vi "Strip Struct Padding.vi"(8 "error in (no error)":errorcluster, 9 "[Sub-Item Type Information]":T1[](array[typedef]), 10 "Byte Stream in":u8[](array[numeric]), 11 "TwinCAT ADS in":refnum<class "TwinCAT ADS.lvclass">) -> (0 "error out":errorcluster, 2 "Data String":string, 3 "TwinCAT ADS out":refnum<class "TwinCAT ADS.lvclass">)   [LabVIEW 2018, in "TwinCAT ADS.lvclass"]
uses:
  TwinCAT ADS.lvclass
  Controls/PLC Sub-Item Type Descriptor.ctl
  Controls/PLC Type.ctl
  Controls/PLC Array Type Descriptor.ctl
  PLC Primitive Byte Stream to Data String.vi/dd5e40b3-f89d-44d0-b911-1f2dc1f1e391.vi
  PLC Primitive Byte Stream to Data String.vi/9a8c356b-cf55-4838-9201-0532b80217b2.vi
  PLC Primitive Byte Stream to Data String.vi/06482052-d1f9-4f29-aca9-908031c6a69f.vi
  PLC Primitive Byte Stream to Data String.vi/b9242781-96b0-446e-9150-452b1084ed54.vi
  PLC Primitive Byte Stream to Data String.vi/5fbe6976-0b86-40a2-b7b6-3748894f0071.vi
  PLC Primitive Byte Stream to Data String.vi/c4de1741-fffd-4fed-ba25-d7b4acbf0555.vi
  PLC Primitive Byte Stream to Data String.vi/20356124-05d2-4a04-a5d1-e69adc4c58c2.vi
  PLC Primitive Byte Stream to Data String.vi/67ddb754-0fbe-43d9-9e61-34d6659124ef.vi
  PLC Primitive Byte Stream to Data String.vi/e3d41cb3-d20e-45e9-8252-e41884a8f4d0.vi
  PLC Primitive Byte Stream to Data String.vi/46ba2a54-cc07-4222-9a0e-bd972edfcef0.vi
  PLC Primitive Byte Stream to Data String.vi/6b416cf7-30dc-48a3-9278-9d800f443678.vi
  PLC Primitive Byte Stream to Data String.vi/5857d013-9824-4299-a2d7-53efdc0d26c5.vi
  PLC Primitive Byte Stream to Data String.vi/006b0e7e-7e80-41f3-be4e-1f3da8479fae.vi
  PLC Primitive Byte Stream to Data String.vi/28d9c90b-5f2a-4c58-95e2-5fc46303b0fd.vi
  PLC Primitive Byte Stream to Data String.vi/99b7bc4a-962e-4818-aa5d-444f23f83b11.vi
  PLC Primitive Byte Stream to Data String.vi/8b7c42c8-9170-4542-8f35-15cbeddc22cb.vi
  PLC Primitive Byte Stream to Data String.vi/65a091fa-0bd2-4a35-ae2b-3fa5e90d1994.vi
  PLC Primitive Byte Stream to Data String.vi/4b7d3a7d-7f1b-46f0-9357-48cb72148c56.vi
  PLC Primitive Byte Stream to Data String.vi/b431183c-2ad5-4c6d-9bfa-a53b18913682.vi
  PLC Primitive Byte Stream to Data String.vi/30c6c28a-53c3-4e33-80b1-b22f521e1f67.vi
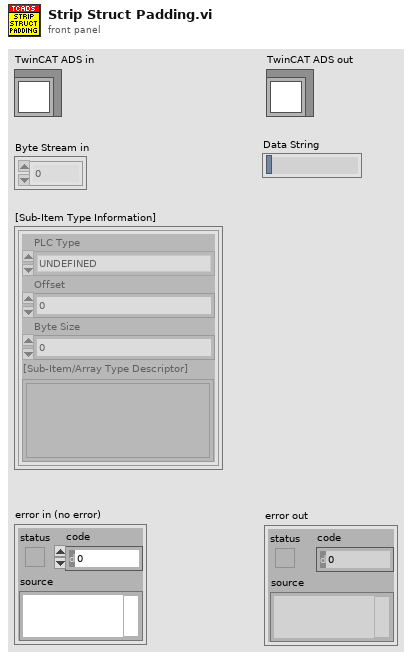
[diagram p1: front panel]
types:
  T1 = typedef "TwinCAT ADS.lvclass/PLC Sub-Item Type Descriptor.ctl" = cluster{"PLC Type":T2, "Offset":i32, "Byte Size":i32, "[Sub-Item/Array Type Descriptor]":variant[]}
  T2 = typedef "TwinCAT ADS.lvclass/PLC Type.ctl" = enum16{"UNDEFINED", "INT", "DINT", "REAL", "LREAL", "SINT", "BYTE", "UINT", "UDINT", "LINT", "ULINT", "STRING", "WSTRING", "BOOL", "TIME", "LTIME", "DATE", "DT", "TOD", "ARRAY", "JAGGED ARRAY", "STRUCT", "FUNCTION BLOCK", "UNION", "POINTER", "USER DEFINED"}
  T3 = typedef "TwinCAT ADS.lvclass/PLC Array Type Descriptor.ctl" = cluster{"Fundamental PLC Type":T2, "Fundamental Type Byte Size":i32, "Item Count":i32, "Dimension Lengths":i32[], "Sub-Item Type Descriptor":variant}
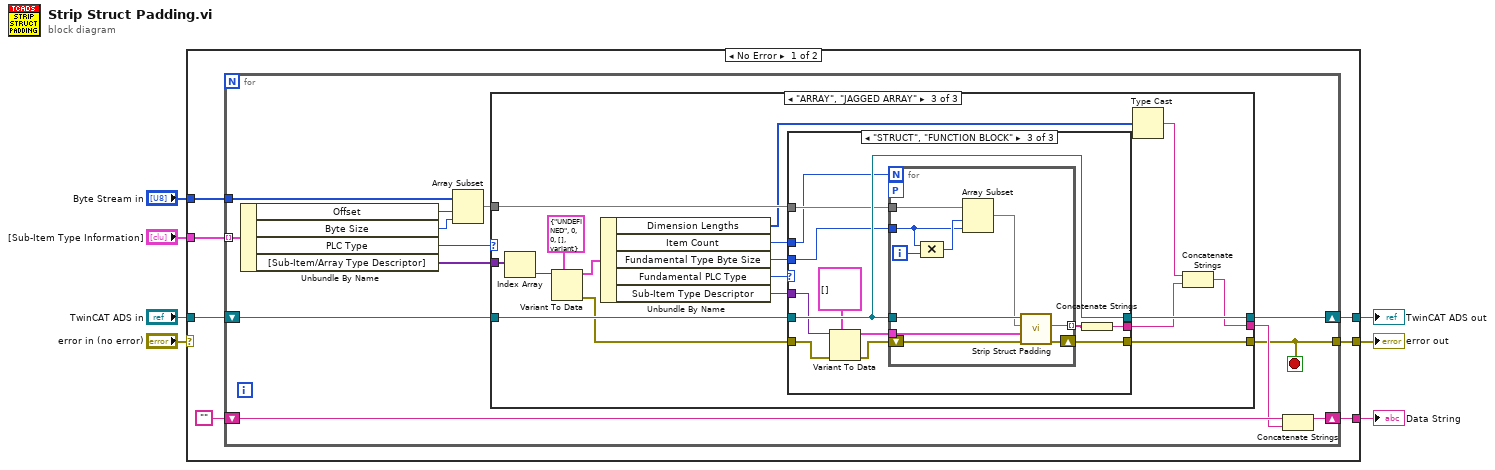
[diagram p0: block diagram]
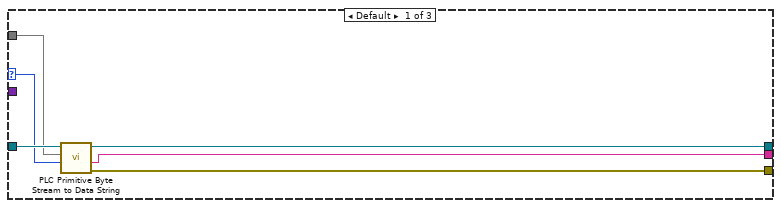
[diagram p2: hidden frame]
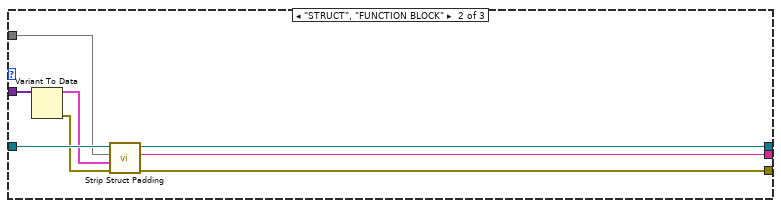
[diagram p3: hidden frame]
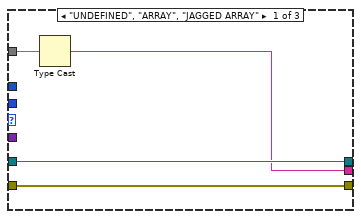
[diagram p4: hidden frame]
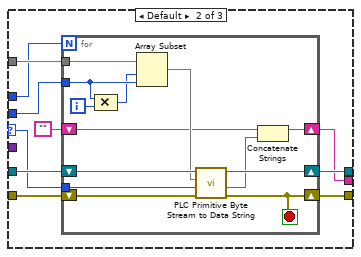
[diagram p5: hidden frame]
diagram:
  n1 = case shown="No Error" "error in (no error)" {
    selector: "error in (no error)" -> [_ w109]
    tunnel: "[Sub-Item Type Information]" -> [w14 _]
    tunnel: "Byte Stream in" -> [w13 _]
    tunnel: [w11 _] -> w5
    tunnel: [w10 w109] -> w4
    tunnel: "TwinCAT ADS in" -> [w9 w108]
    tunnel: [w8 w108] -> w1
    frame No Error {
      n2 = for {
        tunnel: w14 -> [w27] mode=indexing
        shift-right: [w20] -> w11
        shift-left: "" -> [w21]
        tunnel: [w17] -> w10
        tunnel: w13 -> [w26]
        shift-right: [w16] -> w8
        shift-left: w9 -> [w15]
        stop <- w17 stop-if-true
        n3 = Unbundle By Name(w27) -> ("Offset"=w25:i32, "Byte Size"=w24:i32, "PLC Type"=w22:T2, "[Sub-Item/Array Type Descriptor]"=w18:variant[])
        n4 = Array Subset(array=w26, index=w25, length=w24) -> (w23:u8[])
        n5 = case shown="\"ARRAY\", \"JAGGED ARRAY\"" w22 {
          selector: w22 -> [w32 _ _]
          tunnel: w23 -> [w31 w35 w51]
          tunnel: [w28 w37 w42] -> w19
          tunnel: w18 -> [_ w39 w58]
          tunnel: [w30 w38 w45] -> w17
          tunnel: [w29 w34 w46] -> w16
          tunnel: w15 -> [w33 w41 w54]
          frame Default {
            n6 = call "PLC Primitive Byte Stream to Data String.vi"("PLC Type"=w32, "Byte Stream"=w31, "TwinCAT ADS in"=w33) -> ("error out"=w30:errorcluster, "Data String"=w28:string, "TwinCAT ADS out"=w29:refnum<class "TwinCAT ADS.lvclass">)  [unwired: 5 in, 1 out]
          }
          frame "STRUCT", "FUNCTION BLOCK" {
            n7 = Variant To Data(Variant=w39) -> (data=w36:T1[], error out=w40:errorcluster)  [unwired: 2 in]
            n8 = call "Strip Struct Padding.vi"("error in (no error)"=w40, "[Sub-Item Type Information]"=w36, "Byte Stream in"=w35, "TwinCAT ADS in"=w41) -> ("error out"=w38:errorcluster, "Data String"=w37:string, "TwinCAT ADS out"=w34:refnum<class "TwinCAT ADS.lvclass">)  [unwired: 5 in]
          }
          frame "ARRAY", "JAGGED ARRAY" {
            n9 = Index Array(array=w58) -> (element=w57:variant)  [unwired: 1 in]
            n10 = Variant To Data(type=T3 {"Fundamental PLC Type"=enum."UNDEFINED", "Fundamental Type Byte Size"=0, "Item Count"=0, "Dimension Lengths"=[], "Sub-Item Type Descriptor"=variant} ("Array Information"), Variant=w57) -> (data=w55:T3, error out=w52:errorcluster)  [unwired: 1 in]
            n11 = Unbundle By Name(w55) -> ("Dimension Lengths"=w47:i32[], "Item Count"=w48:i32, "Fundamental Type Byte Size"=w49:i32, "Fundamental PLC Type"=w50:T2, "Sub-Item Type Descriptor"=w53:variant)
            n12 = case shown="\"STRUCT\", \"FUNCTION BLOCK\"" w50 {
              selector: w50 -> [_ w66 _]
              tunnel: w52 -> [w61 w67 w92]
              tunnel: w54 -> [w62 w71 w97]
              tunnel: w51 -> [w60 w72 w95]
              tunnel: [w61 w65 w96] -> w45
              tunnel: [w62 w64 w97] -> w46
              tunnel: w53 -> [_ _ w91]
              tunnel: w48 -> [_ w70 w94]
              tunnel: w49 -> [_ w69 w93]
              tunnel: [w59 w63 w86] -> w44
              frame "UNDEFINED", "ARRAY", "JAGGED ARRAY" {
                n13 = Type Cast(x=w60) -> (*(type *) &x=w59:string)  [unwired: 1 in]
              }
              frame Default {
                n14 = for {
                  N: w70 -> [_]
                  shift-right: [w77] -> w64
                  shift-left: w71 -> [w81]
                  tunnel: w66 -> [w79]
                  tunnel: w69 -> [w83]
                  shift-right: [w76] -> w65
                  shift-left: w67 -> [w80]
                  tunnel: w72 -> [w85]
                  shift-right: [w74] -> w63
                  shift-left: "" -> [w73]
                  i -> [w84]
                  stop <- w76 stop-if-true
                  n15 = Compound Arithmetic op=MULTIPLY(w83, w84) -> (w82:i32)
                  n16 = Array Subset(array=w85, index=w82, length=w83) -> (w78:u8[])
                  n17 = call "PLC Primitive Byte Stream to Data String.vi"("error in (no error)"=w80, "PLC Type"=w79, "Byte Stream"=w78, "TwinCAT ADS in"=w81) -> ("error out"=w76:errorcluster, "Data String"=w75:string, "TwinCAT ADS out"=w77:refnum<class "TwinCAT ADS.lvclass">)  [unwired: 4 in, 1 out]
                  n18 = Concatenate Strings(w73, w75) -> (w74:string)
                }
              }
              frame "STRUCT", "FUNCTION BLOCK" {
                n19 = Variant To Data(error in=w92, type=T1[] [] ("[Sub-Item Type Information]"), Variant=w91) -> (data=w88:T1[], error out=w90:errorcluster)
                n20 = for {
                  N: w94 -> [_]
                  tunnel: w93 -> [w104]
                  tunnel: w88 -> [w103]
                  shift-right: [w99] -> w96
                  shift-left: w90 -> [w101]
                  tunnel: w95 -> [w106]
                  workers-P: _ -> [_]
                  tunnel: w97 -> [w102]
                  tunnel: [w100] -> w87 mode=indexing
                  i -> [w105]
                  n21 = Compound Arithmetic op=MULTIPLY(w104, w105) -> (w107:i32)
                  n22 = Array Subset(array=w106, index=w107, length=w104) -> (w98:u8[])
                  n23 = call "Strip Struct Padding.vi"("error in (no error)"=w101, "[Sub-Item Type Information]"=w103, "Byte Stream in"=w98, "TwinCAT ADS in"=w102) -> ("error out"=w99:errorcluster, "Data String"=w100:string)  [unwired: 5 in, 1 out]
                }
                n24 = Concatenate Strings(w87) -> (w86:string)
              }
            }
            n25 = Type Cast(x=w47) -> (*(type *) &x=w43:string)  [unwired: 1 in]
            n26 = Concatenate Strings(w43, w44) -> (w42:string)
          }
        }
        n27 = Concatenate Strings(w21, w19) -> (w20:string)
      }
    }
    frame Error {
    }
  }
  "Data String" <- w5
  "error out" <- w4
  "TwinCAT ADS out" <- w1
